vi "o-scope.vi"() -> ()   [LabVIEW 2009]
panel:
  out "Waveform Graph":dbl[](graph)
  # "items to include:\nvertical shift\nhorizontal shift\namplitude\nplot length\nperiod\nduty cycle"
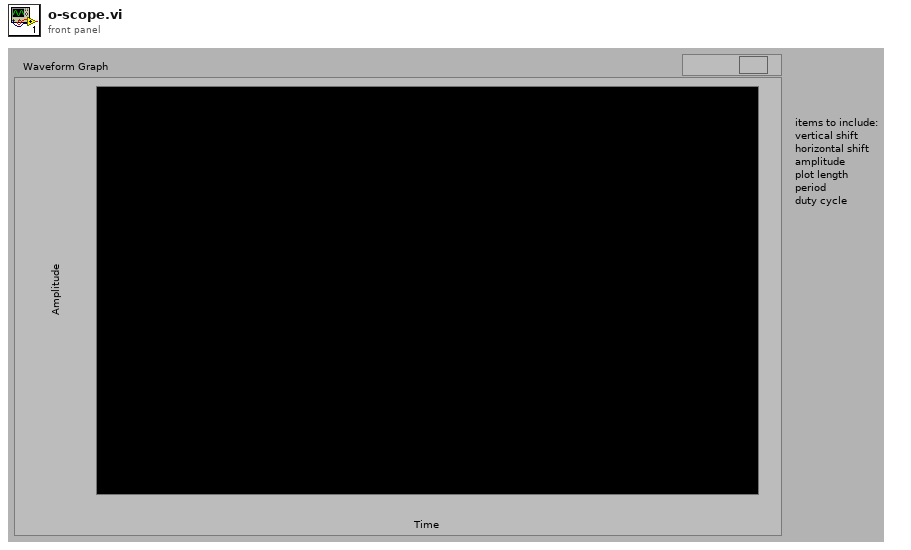
[diagram p1: front panel]
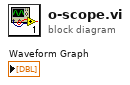
[diagram p0: block diagram]
diagram:
